vi "find sequence.vi"(10 "sequence name":string, 11 "Simple Sequencer TBM configuration in":refnum<class "Simple Sequencer TBM configuration.lvclass">) -> (2 "index":i32, 3 "Simple Sequencer TBM configuration out":refnum<class "Simple Sequencer TBM configuration.lvclass">)   [LabVIEW 2014, in "Simple Sequencer TBM configuration.lvclass"]
uses:
  Simple Sequencer TBM configuration.lvclass
  Simple Sequencer TBM configuration.lvclass/Simple Sequencer TBM configuration.ctl
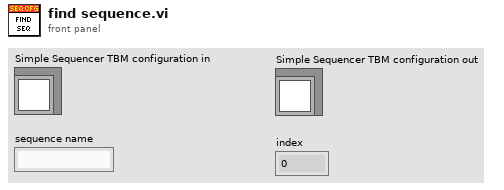
[diagram p1: front panel]
types:
  T1 = typedef "Simple Sequencer TBM configuration.lvclass/sequence definition.ctl" = cluster{"sequence name":string, "action configs":refnum<class "action configuration.lvclass">[]}
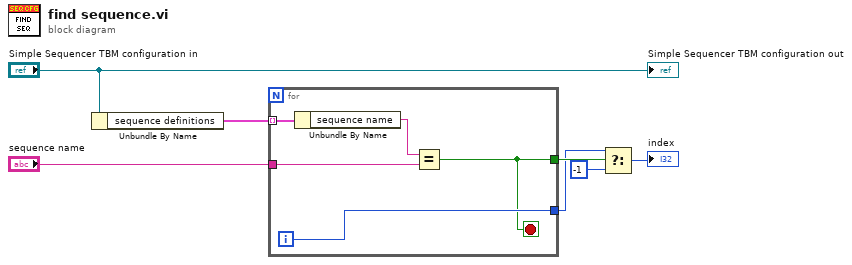
[diagram p0: block diagram]
diagram:
  n1 = Unbundle By Name("Simple Sequencer TBM configuration in") -> ("sequence definitions"=w6:T1[])
  n2 = for {
    tunnel: w6 -> [w12] mode=indexing
    tunnel: "sequence name" -> [w10]
    tunnel: [w9] -> w3
    tunnel: [w8] -> w4
    i -> [w9]
    stop <- w8 stop-if-true
    n3 = Unbundle By Name(w12) -> ("sequence name"=w11:string)
    n4 = Equal?(x=w11, y=w10) -> (x = y?=w8:bool)
  }
  n5 = Select(t=w3, s=w4, f=-1) -> (s? t:f=→"index":i32)
  "Simple Sequencer TBM configuration out" <- "Simple Sequencer TBM configuration in"
